vi "OAT Resample (Const to Variable).vi"(5 "reset? (True)":bool=TRUE, 8 "error in (no error)":errorcluster, 9 "filter prototype":T2={"left wing"=[], "increment"=[], "max dec"=128, "timing jitter"=enum."Interpolation", "band limiting?"=TRUE} {"increment" format="%.2f"; "left wing" format="%.2f"}, 10 "time":dbl[](array[numeric]) format="%.2f", 11 "scaled signals (EU)":waveform(dbl)[](array[waveform])) -> (0 "error out":errorcluster, 1 "offset":dbl, 2 "time stamps":dbl[](array[numeric]) format="%.2f", 3 "Y":dbl[][](array[numeric]) format="%.2f")   [LabVIEW 2017, in "SoundVib_Resampling.lvlib"]
doc: "Perform an arbitrary resampling on the input signal."
uses:
  <vilib>/addons/Sound and Vibration/Order Analysis/Resample Order Tracking/SoundVib_Resampling.lvlib
  <vilib>/addons/_NISVFA/_Shared subVIs/Controls/OAT Resample Filter Prototype.ctl
  <resource>/sndvib.dll
panel:
  in  "state in":T1 {"time interval" format="%.2f"; "position" format="%.2f"; "init condition" format="%.2f"}
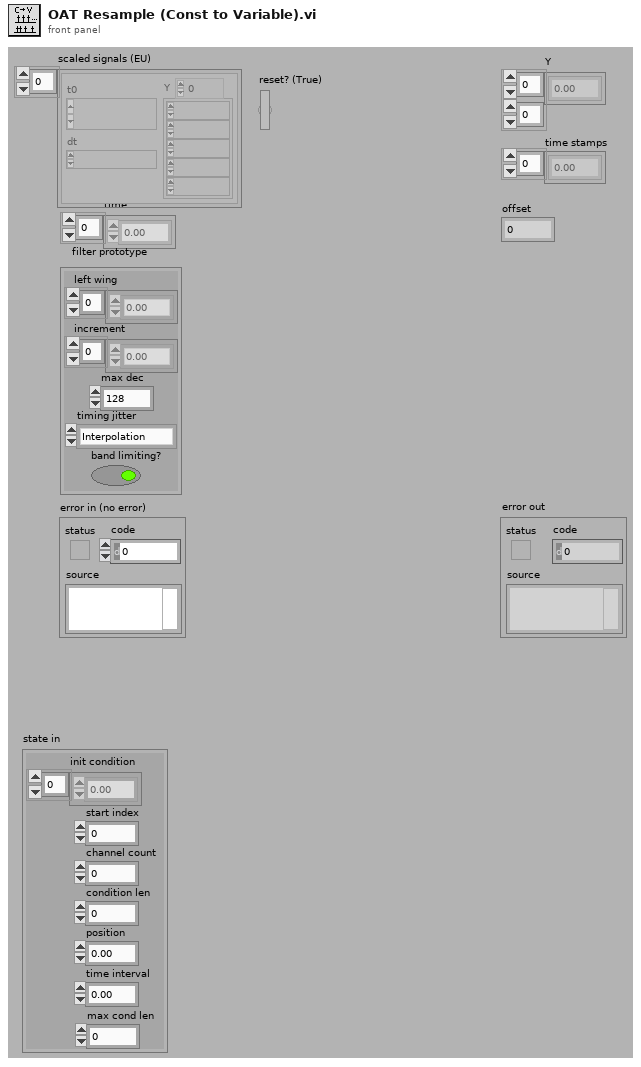
[diagram p1: front panel]
types:
  T1 = cluster{"init condition":dbl[], "start index":i32, "channel count":i32, "condition len":i32, "position":dbl, "time interval":dbl, "max cond len":i32}
  T2 = typedef "OAT Resample Filter Prototype.ctl" = cluster{"left wing":dbl[], "increment":dbl[], "max dec":i32, "timing jitter":enum32{"Interpolation", "Rounding"}, "band limiting?":bool}
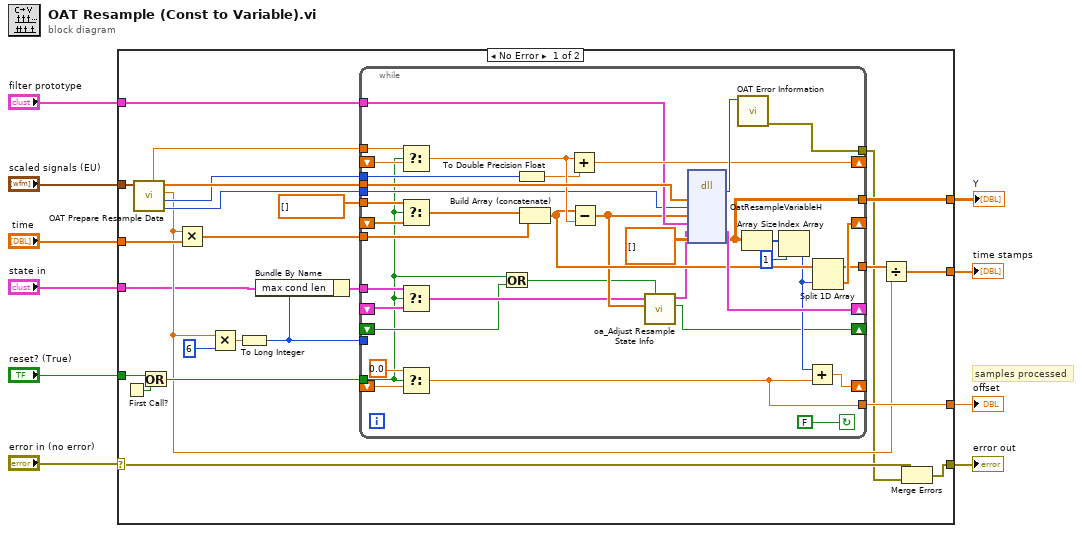
[diagram p0: block diagram]
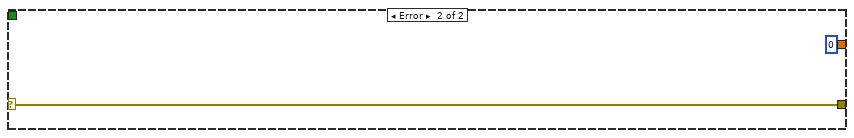
[diagram p2: hidden frame]
diagram:
  # "samples processed"
  n1 = case shown="No Error" "error in (no error)" {
    selector: "error in (no error)" -> [w15 w75]
    tunnel: "filter prototype" -> [w35 _]
    tunnel: "time" -> [w34 _]
    tunnel: [w31 _] -> w8
    tunnel: [w29 0] -> w7
    tunnel: [w13 w75] -> w6
    tunnel: "scaled signals (EU)" -> [w32 _]
    tunnel: [w25 _] -> w3
    tunnel: "reset? (True)" -> [w22 _]
    tunnel: "state in" -> [w11 _]
    frame No Error {
      n2 = First Call?() -> (First Call?: T/F=w23:bool)
      n3 = call <vilib>:"OAT Prepare Resample Data.vi"("Array"=w32) -> ("channel count"=w26:i32, "signal len"=w28:i32, "fs"=w20:dbl, "Y"=w33:dbl[], "elapsed length"=w12:dbl)  [unwired: 6 in]
      n4 = Or(x=w22, y=w23) -> (x .or. y?=w21:bool)
      n5 = Multiply(x=w20, y=w34) -> (x*y=w24:dbl[])
      n6 = Multiply(x=w20, y=6) -> (x*y=w18:dbl)
      n7 = To Long Integer(number=w18) -> (32bit integer=w17:i32)
      n8 = Bundle By Name(cluster=w11, "max cond len"=w17) -> (w16:T1)
      n9 = while {
        shift-right: [w54] -> _
        shift-left: _ -> [w66]
        tunnel: w33 -> [w69]
        tunnel: w24 -> [w68]
        shift-right: [w64] -> _
        shift-left: _ -> [w70]
        tunnel: w21 -> [w37]
        tunnel: w35 -> [w55]
        shift-right: [w60] -> _
        shift-left: _ -> [w62]
        tunnel: [w71] -> w14
        tunnel: [w41] -> w31
        tunnel: w16 -> [w67]
        tunnel: dbl[] [] ("t") -> [w63]
        tunnel: [w52] -> w27
        tunnel: [w58] -> w29
        shift-right: [w56] -> _
        shift-left: _ -> [w59]
        tunnel: w28 -> [w51]
        tunnel: w26 -> [w53]
        tunnel: w17 -> [_]
        tunnel: w12 -> [w40]
        shift-right: [w39] -> _
        shift-left: _ -> [w38]
        stop <- FALSE continue-if-true
        n10 = Select(t=w40, s=w37, f=w59) -> (s? t:f=w57:dbl)
        n11 = Select(t=w63, s=w37, f=w70) -> (s? t:f=w65:dbl[])
        n12 = Select(t=w67, s=w37, f=w66) -> (s? t:f=w43:T1)
        n13 = Select(t=0.0, s=w37, f=w62) -> (s? t:f=w58:dbl)
        n14 = Or(x=w37, y=w38) -> (x .or. y?=w36:bool)
        n15 = To Double Precision Float(number=w51) -> (double precision float=w50:dbl)
        n16 = Build Array (concatenate)(w65, w68) -> (w49:dbl[])
        n17 = Add(x=w57, y=w50) -> (x+y=w56:dbl)
        n18 = Subtract(x=w49, y=w57) -> (x-y=w44:dbl[])
        n19 = call <vilib>:"oa_Adjust Resample State Info.vi"("Reset? (True)"=w36, "time position"=w44, "state in"=w43) -> ("reset pending"=w39:bool, "state out"=w42:T1)  [unwired: 7 in]
        n20 = dll-call lib="C:/Program Files (x86)/National Instruments/LabVIEW 2017/resource/sndvib.*" fn="OatResampleVariableH"("signalH"=w69, "channelCount"=w53, "timeH"=w44, "prototype"=w55, "state"=w42, "yH"=dbl[][] []) -> ("return type"=w72:i32, "state"=w54:T1, "yH"=w41:dbl[][])  [unwired: 7 in, 2 out]
        n21 = call <vilib>:"OAT Error Information.vi"("error code"=w72) -> ("error out"=w71:errorcluster)  [unwired: 6 in]
        n22 = Array Size(array=w41) -> (size(s)=w47:i32[])
        n23 = Index Array(array=w47, index=1) -> (element=w45:i32)
        n24 = Add(x=w45, y=w58) -> (x+y=w60:dbl)
        n25 = Split 1D Array(array=w49, index=w45) -> (first subarray=w52:dbl[], second subarray=w64:dbl[])
      }
      n26 = Divide(x=w27, y=w20) -> (x/y=w25:dbl[])
      n27 = Merge Errors(w15, w14) -> (w13:errorcluster)
    }
    frame Error {
    }
  }
  "time stamps" <- w3
  "Y" <- w8
  "offset" <- w7
  "error out" <- w6
